vi "detObjects.vi"(2 "error in (no error)":errorcluster, 3 "Image in":T1) -> (0 "error out":errorcluster, 1 "Output":i32)   [LabVIEW 2009, in "Main.lvlib"]
uses:
  Main.lvlib
  <vilib>/vision/Image Controls.llb/IMAQ Image.ctl
  <vilib>/vision/NI_Vision_Development_Module.lvlib
panel:
  out "Objects":T1(plugin-control)
  out "Number of Objects":i32
  out "Blue layer":T1(plugin-control)
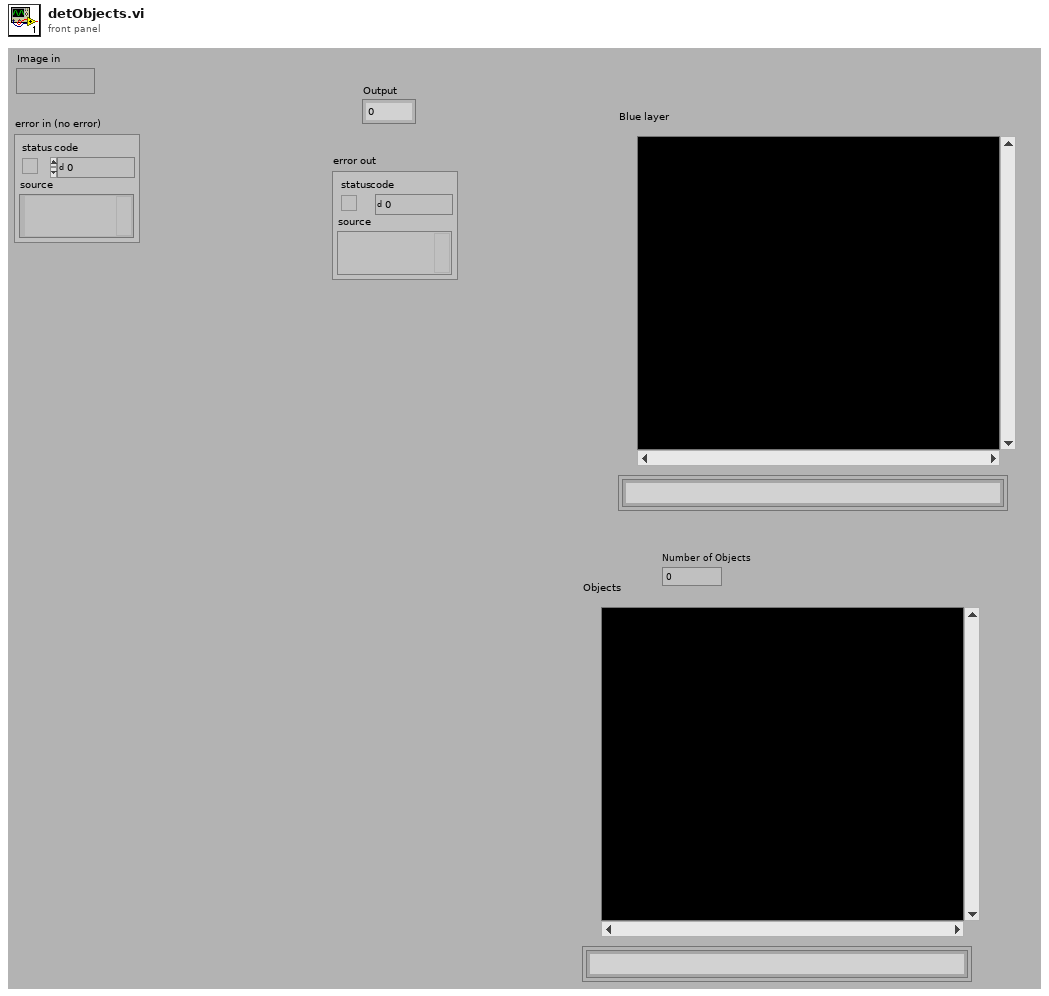
[diagram p1: front panel]
types:
  T1 = typedef "IMAQ Image.ctl" = refnum<image>
  T2 = cluster{"Objects":u16, "Threshold":i32, "Reject Border":bool, "Fill Holes":bool, "Min Object Size":bool, "Min Size":i32, "Max Object Size":bool, "Max Size":i32, "Show Search Area":bool, "Show Center":bool, "Show Bounding Box":bool}
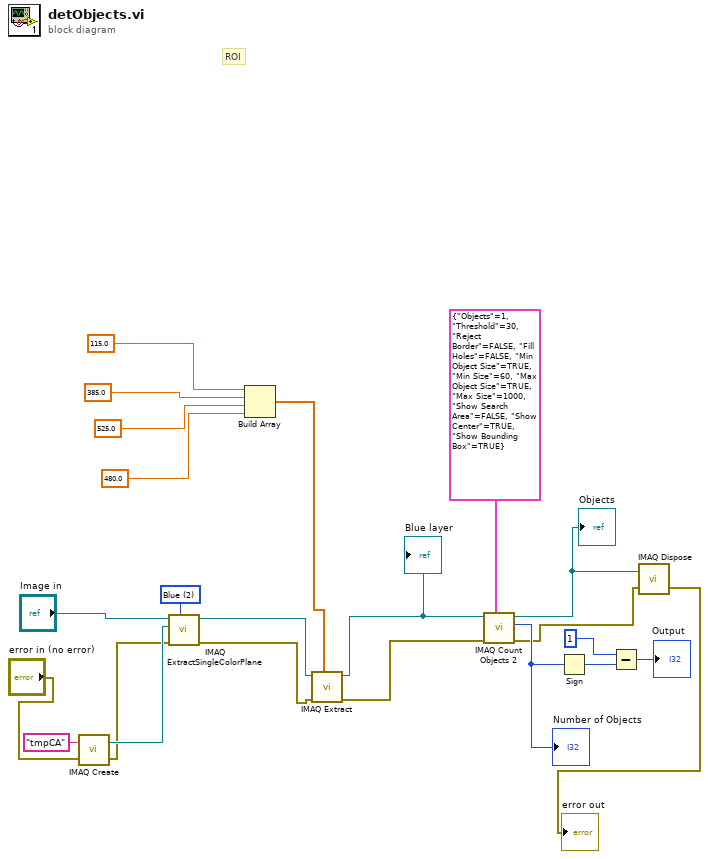
[diagram p0: block diagram]
diagram:
  w23 = 2 items=["Red", "Green", "Blue", "Hue", "Saturation", "Luminance", "Value", "Intensity"] ("Color Plane")
  # "ROI"
  n1 = call "IMAQ Create"("Image Name"="tmpCA", "error in (no error)"="error in (no error)") -> ("New Image"=w6:T1, "error out"=w4:errorcluster)  [unwired: 3 in]
  n2 = call "IMAQ ExtractSingleColorPlane"("Color Plane"=w23, "error in (no error)"=w4, "Image Dst"=w6, "Image Src"="Image in") -> ("error out"=w9:errorcluster, "Image Dst Out"=w13:T1)  [unwired: 6 in]
  n3 = Build Array(115.0 ("element"), 385.0 ("element"), 525.0 ("element"), 480.0 ("element")) -> (w11:dbl[])
  n4 = call "IMAQ Extract"("Optional Rectangle"=w11, "error in (no error)"=w9, "Image Src"=w13) -> ("error out"=w8:errorcluster, "Image Dst Out"=w12:T1)  [unwired: 7 in]
  "Blue layer" <- w12
  n5 = call "IMAQ Count Objects 2"("Settings"=T2 {"Objects"=1, "Threshold"=30, "Reject Border"=FALSE, "Fill Holes"=FALSE, "Min Object Size"=TRUE, "Min Size"=60, "Max Object Size"=TRUE, "Max Size"=1000, "Show Search Area"=FALSE, "Show Center"=TRUE, "Show Bounding Box"=TRUE}, "error in (no error)"=w8, "Image"=w12) -> ("error out"=w2:errorcluster, "Number of Objects"=w22:i32, "Image Out"=w3:T1)  [unwired: 4 in, 2 out]
  "Number of Objects" <- w22
  "Objects" <- w3
  n6 = Sign(1:w22) -> (0:w21:i32)
  n7 = Subtract(x=1, y=w21) -> (x-y=→"Output":i32)
  n8 = call "IMAQ Dispose"("Image"=w3, "error in (no error)"=w2) -> ("error out"=→"error out":errorcluster)  [unwired: 4 in]
